vi "Extract Multiple Tone Information N Chan.vi"(0 "time signals in":waveform(dbl)[](array[waveform]), 5 "export mode":T3(ring), 7 "threshold":dbl=0.001 format="%#_6p", 9 "max num tones":i32=4, 11 "error in (no error)":errorcluster, 12 "output sorting":i32(ring) items=["increasing frequency", "decreasing amplitude"]) -> (3 "exported signals":T2(array[cluster]) {"exported spectrum (dB)"."dB Spectrum (Hann)" format="%.2p"; "exported spectrum (dB)"."df" format="%.2p"; "exported spectrum (dB)"."f0" format="%.2p"}, 4 "multiple tone information":T1(array[cluster]) {"multiple tone information"."detected phase (deg)" format="%_6g"; "multiple tone information"."detected amplitude" format="%_6p"; "multiple tone information"."detected frequency" format="%_6p"}, 15 "error out":errorcluster)   [LabVIEW 2020, in "NI_MAPro.lvlib"]
doc: "Returns the frequency, amplitude, and phase for each signal tone whose amplitude exceeds a specified <B>threshold</B>. Wire data to the <B>time signal in</B> input to determine the polymorphic instance to use or manually select the instance."
uses:
  NI_MAPro.lvlib
  NI_MABase.lvlib
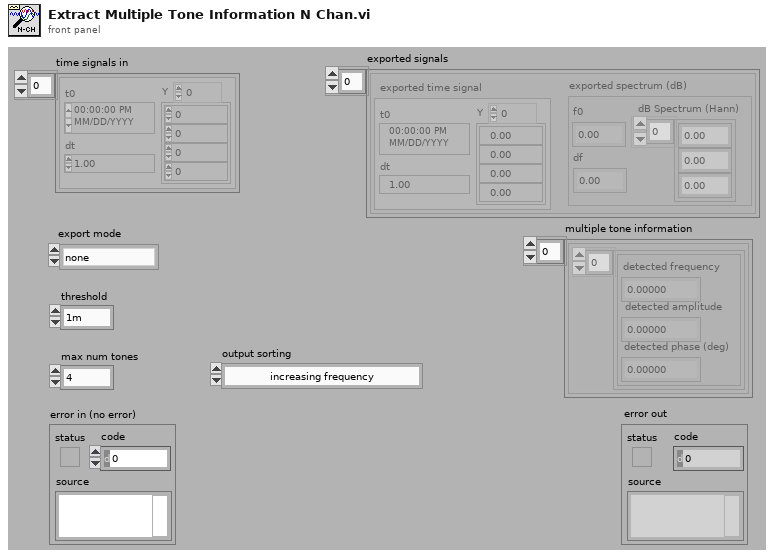
[diagram p1: front panel]
types:
  T1 = cluster{"multiple tone information":cluster{"detected frequency":dbl, "detected amplitude":dbl, "detected phase (deg)":dbl}[]}[]
  T2 = cluster{"exported time signal":waveform(dbl), "exported spectrum (dB)":cluster{"f0":dbl, "df":dbl, "dB Spectrum (Hann)":dbl[]}}[]
  T3 = enum32{"none", "input signal", "detected signal", "residual signal"}
  T4 = cluster{"exported time signal":waveform(dbl), "exported spectrum (dB)":cluster{"f0":dbl, "df":dbl, "dB Spectrum (Hann)":dbl[]}}
  T5 = cluster{"detected frequency":dbl, "detected amplitude":dbl, "detected phase (deg)":dbl}[]
  T6 = cluster{"multiple tone information":cluster{"detected frequency":dbl, "detected amplitude":dbl, "detected phase (deg)":dbl}[]}
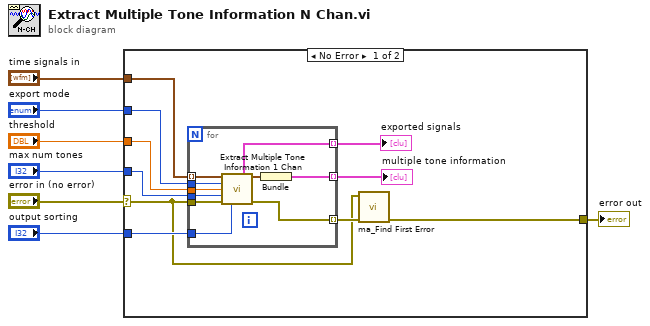
[diagram p0: block diagram]
diagram:
  n1 = case shown="No Error" "error in (no error)" {
    selector: "error in (no error)" -> [w10 w28]
    tunnel: "max num tones" -> [w17 _]
    tunnel: "threshold" -> [w16 _]
    tunnel: "export mode" -> [w15 _]
    tunnel: "output sorting" -> [w14 _]
    tunnel: "time signals in" -> [w13 _]
    tunnel: [w11 w28] -> w2
    frame No Error {
      n2 = for {
        tunnel: w10 -> [w27]
        tunnel: w17 -> [w26]
        tunnel: w16 -> [w25]
        tunnel: w15 -> [w24]
        tunnel: w14 -> [w23]
        tunnel: w13 -> [w22] mode=indexing
        tunnel: [w21] -> w9 mode=indexing
        tunnel: [w19] -> w8 mode=indexing
        tunnel: [w18] -> w12 mode=indexing
        n3 = call "Extract Multiple Tone Information 1 Chan.vi"("time signal in"=w22, "export mode"=w24, "threshold"=w25, "max num tones"=w26, "error in (no error)"=w27, "output sorting"=w23) -> ("exported signals"=w21:T4, "multiple tone information"=w20:T5, "error out"=w18:errorcluster)  [unwired: 7 out]
        n4 = Bundle("multiple tone information"=w20) -> (w19:T6)  [unwired: 1 in]
      }
      "exported signals" <- w9
      "multiple tone information" <- w8
      n5 = call "ma_Find First Error.vi"("error array in"=w12, "error in 1 (no error)"=w10) -> ("error out"=w11:errorcluster)  [unwired: 2 in, 3 out]
    }
    frame Error {
    }
  }
  "error out" <- w2
